vi "OSICS_Wait for message RS232.vi"(8 "error in":errorcluster, 10 "Timeout (s)":sgl=60.0, 11 "VISA IN":refnum<visa-resource-name>) -> (0 "error out":errorcluster, 1 "Returned Message":string, 2 "ERR":i32, 3 "VISA OUT":refnum<visa-resource-name>)   [LabVIEW 2014, in "OSICS_LIB.lvlib"]
doc: "This Vi waits for a message from the COM port until it becomes available or time out is reached, whichever comes first.\nThe obtained message is returned, along with an ERR if an Error has occured.\n\nRS232 only."
uses:
  OSICS_LIB.lvlib
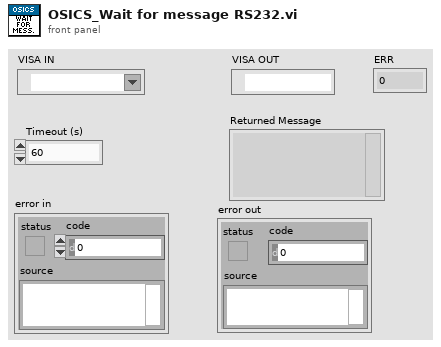
[diagram p1: front panel]
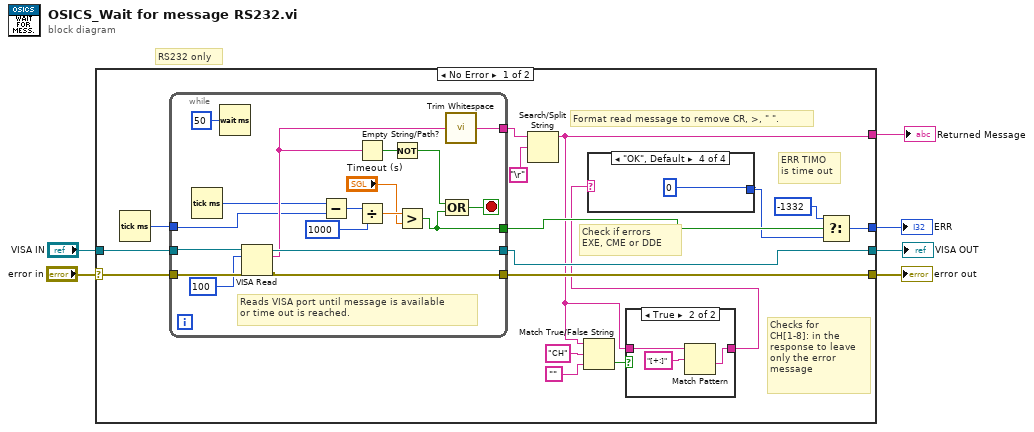
[diagram p0: block diagram]
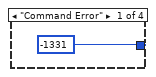
[diagram p2: hidden frame]
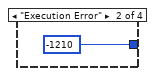
[diagram p3: hidden frame]
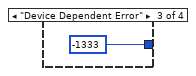
[diagram p4: hidden frame]
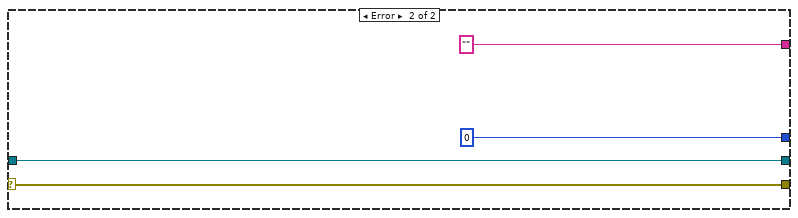
[diagram p6: hidden frame]
diagram:
  # "RS232 only"
  n1 = case shown="No Error" "error in" {
    selector: "error in" -> [w21 w52]
    tunnel: "VISA IN" -> [w22 w51]
    tunnel: [w19 w52] -> w6
    tunnel: [w20 w51] -> w5
    tunnel: [w17 0 ("f")] -> w3
    tunnel: [w10 "" ("Returned Message")] -> w2
    frame No Error {
      # "Checks for \nCH[1-8]: in the\nresponse to leave\nonly the error\nmessage"
      # "ERR TIMO\nis time out"
      # "Check if errors\nEXE, CME or DDE"
      # "Format read message to remove CR, >, \" \"."
      n2 = Tick Count (ms)() -> (millisecond timer value=w7:u32)
      n3 = while {
        tunnel: w22 -> [w47]
        tunnel: w21 -> [w44]
        tunnel: [w45] -> w19
        tunnel: [w46] -> w20
        tunnel: [w32] -> w18
        tunnel: [w38] -> w14
        tunnel: w7 -> [w36]
        stop <- w48 stop-if-true
        # "Reads VISA port until message is available\nor time out is reached."
        n4 = Tick Count (ms)() -> (millisecond timer value=w37:u32)
        n5 = Wait (ms)(milliseconds to wait=u32 50) -> ()  [unwired: 1 out]
        n6 = VISA Read(VISA resource name=w47, byte count=u32 100, error in (no error)=w44) -> (VISA resource name out=w46:refnum<visa-resource-name>, read buffer=w39:string, error out=w45:errorcluster)  [unwired: 1 out]
        n7 = Subtract(x=w37, y=w36) -> (x-y=w35:u32)
        n8 = Empty String/Path?(string/path=w39) -> (empty?=w43:bool)
        n9 = Divide(x=w35, y=u32 1000) -> (x/y=w33:dbl)
        n10 = Not(x=w43) -> (.not. x?=w42:bool)
        n11 = Greater?(x=w33, y="Timeout (s)") -> (0:w32:bool)
        n12 = call <vilib>:"Trim Whitespace.vi"("string"=w39) -> ("trimmed string"=w38:string)  [unwired: 1 in]
        n13 = Compound Arithmetic op=OR(w42, w32) -> (w48:bool)
      }
      n14 = Search/Split String(string=w14, search string/char (-)="\r") -> (substring before match=w10:string)  [unwired: 1 in, 2 out]
      n15 = Match True/False String(2:"", 3:"CH" ("true string"), 4:w10) -> (0:w11:bool)  [unwired: 1 out]
      n16 = case shown="True" w11 {
        tunnel: w10 -> [w27 w29]
        tunnel: [w27 w28] -> w8
        frame False {
        }
        frame True {
          n17 = Match Pattern(string=w29, regular expression="[+:]") -> (after substring=w28:string)  [unwired: 1 in, 3 out]
        }
      }
      n18 = case shown="\"OK\", Default" w8 {
        tunnel: [-1331 -1210 -1333 0 ("f")] -> w9
        frame "Command Error" {
        }
        frame "Execution Error" {
        }
        frame "Device Dependent Error" {
        }
        frame "OK", Default {
        }
      }
      n19 = Select(t=-1332, s=w18, f=w9) -> (s? t:f=w17:i32)
    }
    frame Error {
    }
  }
  "error out" <- w6
  "VISA OUT" <- w5
  "ERR" <- w3
  "Returned Message" <- w2
